vi "WriteDigitalPin.vi"(8 "error in (no error)":errorcluster, 9 "Value":bool, 10 "Pin":T1=2 items=["D2"=2, "D3"=3, "D4"=4, "D5"=5, "D6"=6, "D7"=7, "D8"=8, "D9"=9, "A0"=14, "A1"=15, "A2"=16, "A3"=17], 11 "GrovePi in":refnum<class "GrovePi.lvclass">) -> (0 "error out":errorcluster, 3 "GrovePi out":refnum<class "GrovePi.lvclass">)   [LabVIEW 2014, in "GrovePi.lvclass"]
doc: "Sets the Value of a digital Pin on the GrovePi."
uses:
  GrovePi.lvclass
  Pin.ctl
  Command.ctl
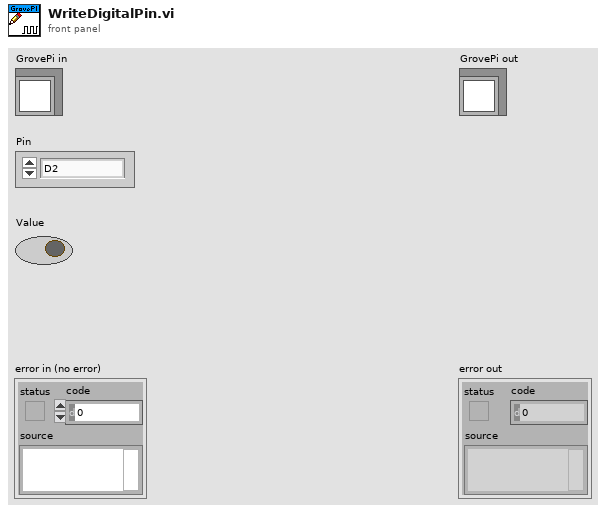
[diagram p1: front panel]
types:
  T1 = typedef "GrovePi.lvclass/Pin.ctl" = u8
  T2 = typedef "GrovePi.lvclass/Command.ctl" = u8
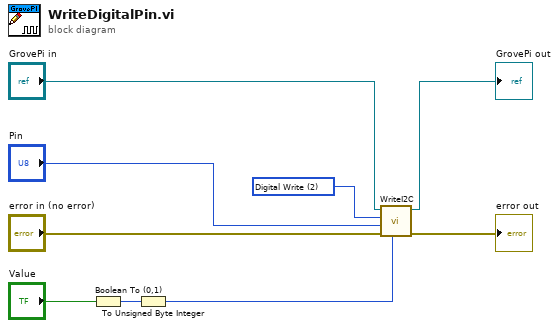
[diagram p0: block diagram]
diagram:
  w2 = T2 2 items=["Digital Read"=1, "Digital Write"=2, "Analog Read"=3, "Analog Write"=4, "Pin Mode"=5, "Ultrasonic Read"=7, "Version"=8, "Dust Sensor Read"=10, "Encoder Read"=11, "Flow Read"=12, "Flow Disabled"=13, "Dust Sensor Enable"=14, "Dust Sensor Disable"=15, "Encoder Enable"=16, "Encoder Disable"=17, "Flow Enable"=18, "Accelerometer Read"=20, "RTC Read"=30, "DHT Read"=40] ("Command")
  n1 = Boolean To (0,1)(Boolean="Value") -> (0, 1=w4:i16)
  n2 = To Unsigned Byte Integer(number=w4) -> (unsigned 8bit integer=w1:u8)
  n3 = call "WriteI2C.vi"("Byte 2"=w1, "error in (no error)"="error in (no error)", "Pin"="Pin", "Command"=w2, "GrovePi in"="GrovePi in") -> ("error out"=→"error out":errorcluster, "GrovePi out"=→"GrovePi out":refnum<class "GrovePi.lvclass">)  [unwired: 4 in, 1 out]
